vi "Functional Global - Configure Test Parameters.vi"(7 "Configure Test Method":T2, 8 "error in (no error)":errorcluster, 11 "Paramater Definition File Path":path) -> (0 "error out":errorcluster, 2 "Experiment Parameter Values":T1(array[cluster]))   [LabVIEW 2014, in "Core SubVIs.lvlib"]
uses:
  Core SubVIs.lvlib
  Controls/TYPE - Configure Test Method.ctl
  <vilib>/Utility/error.llb/DialogType.ctl
  Instance           1 53Saved   Functional Global - Configure Test Parameters .vi
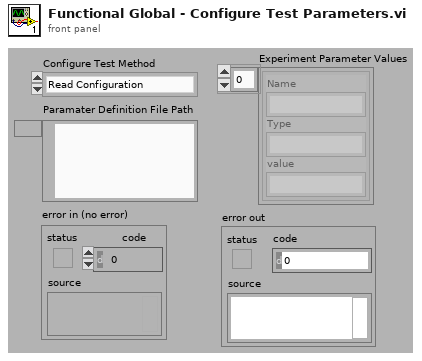
[diagram p1: front panel]
types:
  T1 = cluster{"Name":string, "Type":string, "value":string}[]
  T2 = typedef "Core SubVIs.lvlib/TYPE - Configure Test Method.ctl" = enum16{"Read Configuration", "Load Configuration from File", "Load from default file", "Configuration Dialog"}
  T3 = typedef "DialogType.ctl" = u16
  T4 = cluster{"String":string, "Type":string, "value":string}[]
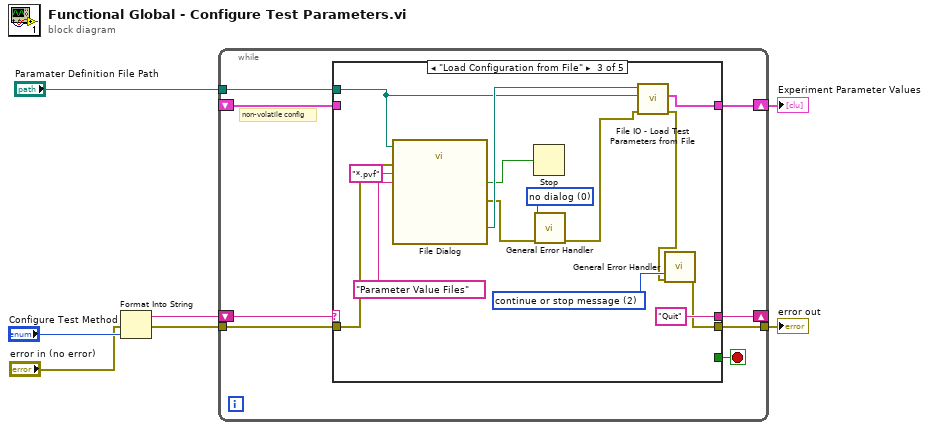
[diagram p0: block diagram]
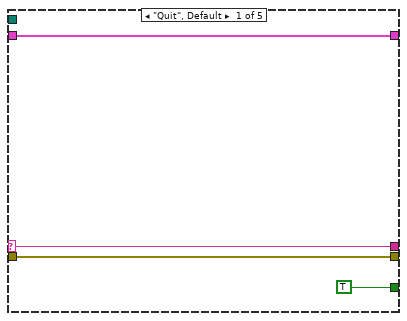
[diagram p2: hidden frame]
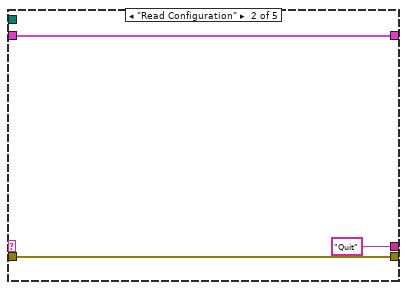
[diagram p3: hidden frame]
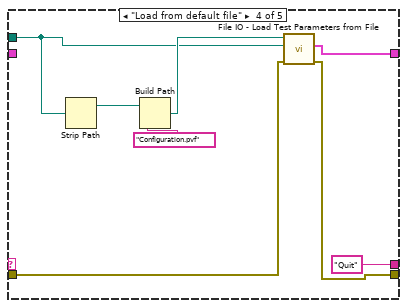
[diagram p4: hidden frame]
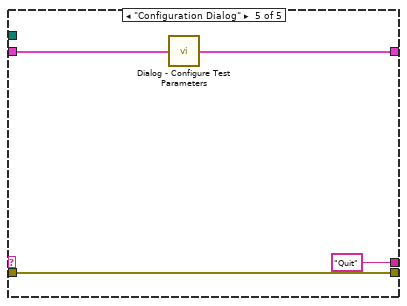
[diagram p5: hidden frame]
diagram:
  n1 = Format Into String(error in="error in (no error)", "Configure Test Method") -> (resulting string=w6:string, error out=w3:errorcluster)  [unwired: 2 in]
  n2 = while {
    shift-right: [w14] -> w1
    shift-left: _ -> [w13]
    shift-right: [w12] -> _
    shift-left: w6 -> [w15]
    tunnel: "Paramater Definition File Path" -> [w10]
    tunnel: w3 -> [w9]
    tunnel: [w8] -> w2
    stop <- w11 stop-if-true
    # "non-volatile config"
    n3 = case shown="\"Load Configuration from File\"" w15 {
      selector: w15 -> [w18 _ _ _ _]
      tunnel: [w19 w22 w35 w41 w45] -> w14
      tunnel: w13 -> [w19 w22 _ _ w46]
      tunnel: [w18 "Quit" "Quit" "Quit" "Quit"] -> w12
      tunnel: [TRUE _ _ _ _] -> w11
      tunnel: w10 -> [_ _ w31 w37 _]
      tunnel: w9 -> [w16 w20 w26 w43 w47]
      tunnel: [w16 w20 w24 w42 w47] -> w8
      frame "Quit", Default {
      }
      frame "Read Configuration" {
      }
      frame "Load Configuration from File" {
        w29 = T3 2 items=["no dialog", "OK message", "continue or stop message", "OK message + warnings", "continue/stop + warnings"] ("type of dialog (OK msg:1)")
        w30 = T3 0 items=["no dialog", "OK message", "continue or stop message", "OK message + warnings", "continue/stop + warnings"] ("type of dialog (OK msg:1)")
        n4 = call "File Dialog"("start path"=w31, "error in"=w26, "pattern (all files)"="*.pvf", "pattern label"="Parameter Value Files") -> ("selected path"=w32:path, "cancelled"=w23:bool, "error out"=w28:errorcluster)  [unwired: 3 in, 6 out]
        n5 = Stop(stop? (T)=w23) -> ()
        n6 = call <vilib>:"General Error Handler.vi"("type of dialog (OK msg:1)"=w30, "error in (no error)"=w28) -> ("error out"=w27:errorcluster)  [unwired: 1 in, 12 out]
        n7 = call "File IO - Load Test Parameters from File.vi"("error in (no error)"=w27, "Parameter Definition File"=w31, "Paramater Value File"=w32) -> ("error out"=w25:errorcluster, "Experiment Parameter Values"=w35:T4)  [unwired: 1 in, 6 out]
        n8 = call <vilib>:"General Error Handler.vi"("type of dialog (OK msg:1)"=w29, "error in (no error)"=w25) -> ("error out"=w24:errorcluster)  [unwired: 1 in, 12 out]
      }
      frame "Load from default file" {
        n9 = Strip Path(path=w37) -> (stripped path=w39:path)  [unwired: 1 out]
        n10 = Build Path(base path=w39, name or relative path="Configuration.pvf") -> (appended path=w38:path)
        n11 = call "File IO - Load Test Parameters from File.vi"("error in (no error)"=w43, "Parameter Definition File"=w37, "Paramater Value File"=w38) -> ("error out"=w42:errorcluster, "Experiment Parameter Values"=w41:T4)  [unwired: 1 in, 6 out]
      }
      frame "Configuration Dialog" {
        n12 = call "Dialog - Configure Test Parameters.vi"("Experiment Parameter Values (default)"=w46) -> ("Experiment Parameter Values (default) 2"=w45:T1)
      }
    }
  }
  "error out" <- w2
  "Experiment Parameter Values" <- w1
